vi "Get Step Number.vi"(11 "Tree Tag":string) -> (1 "Is Step tag?":bool, 2 "Step tag":string, 3 "Step Number":i32)   [LabVIEW 2024, in "Output Sequencer.lvlib" / "Settings UI.lvclass"]
uses:
  Settings UI.lvclass
  Types/Tree Index Enum.ctl
  Globals/Global Tree Data.vi
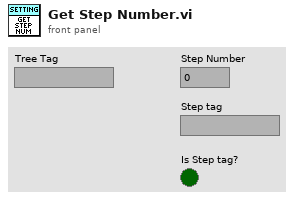
[diagram p1: front panel]
types:
  T1 = typedef "Output Sequencer.lvlib/Settings UI.lvclass/Tree Index Enum.ctl" = enum16{"General Settings", "Num Steps", "Num Analog", "Num Digital", "Show Confirmation", "Interp Priority", "Adv Timing", "Enable Conditions", "Seq Execution", "Reset Test Start", "Only When Test", "Delay After Test", "Start condition", "Re-triggering", "Stop condition", "Stop After Cycles", "Stop Values", "Default Values", "Default Analog", "Default Digital", "Steps", "Step #", "Description", "Precondition", "Duration", "Mode", "Delay Between Vals", "Analog Values", "Digital Values", "Postcondition", "On True", "On False"}
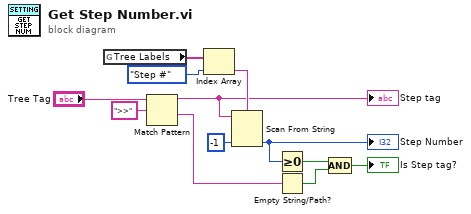
[diagram p0: block diagram]
diagram:
  n1 = global read "Global Tree Data.vi" "Tree Labels"() -> (w10:string[])
  n2 = Match Pattern(string="Tree Tag", regular expression=">>") -> (before substring=w2:string, after substring=w6:string)  [unwired: 1 in, 2 out]
  "Step tag" <- w2
  n3 = Index Array(array=w10, index=Tree_Index_Enum."Step #" ("Tree Index Enum")) -> (element=w8:string)
  n4 = Scan From String(format string=w8, input string=w2, default 1=-1) -> (output 1=w7:i32)  [unwired: 2 in, 3 out]
  "Step Number" <- w7
  n5 = Greater Or Equal To 0?(x=w7) -> (x >= 0?=w5:bool)
  n6 = Empty String/Path?(string/path=w6) -> (empty?=w3:bool)
  n7 = Compound Arithmetic op=AND(w5, w3) -> (→"Is Step tag?":bool)
